vi "桶探测器值数据准备.vi"(0 "模块选择簇":T3, 5 "光源散斑簇":T2, 7 "图像簇":T1) -> (4 "照射差分求和数组":dbl[](array[numeric]), 6 "照射差分求和均值":dbl, 8 "优化光源散斑簇":T2, 10 "优化图像簇":T1)   [LabVIEW 2018]
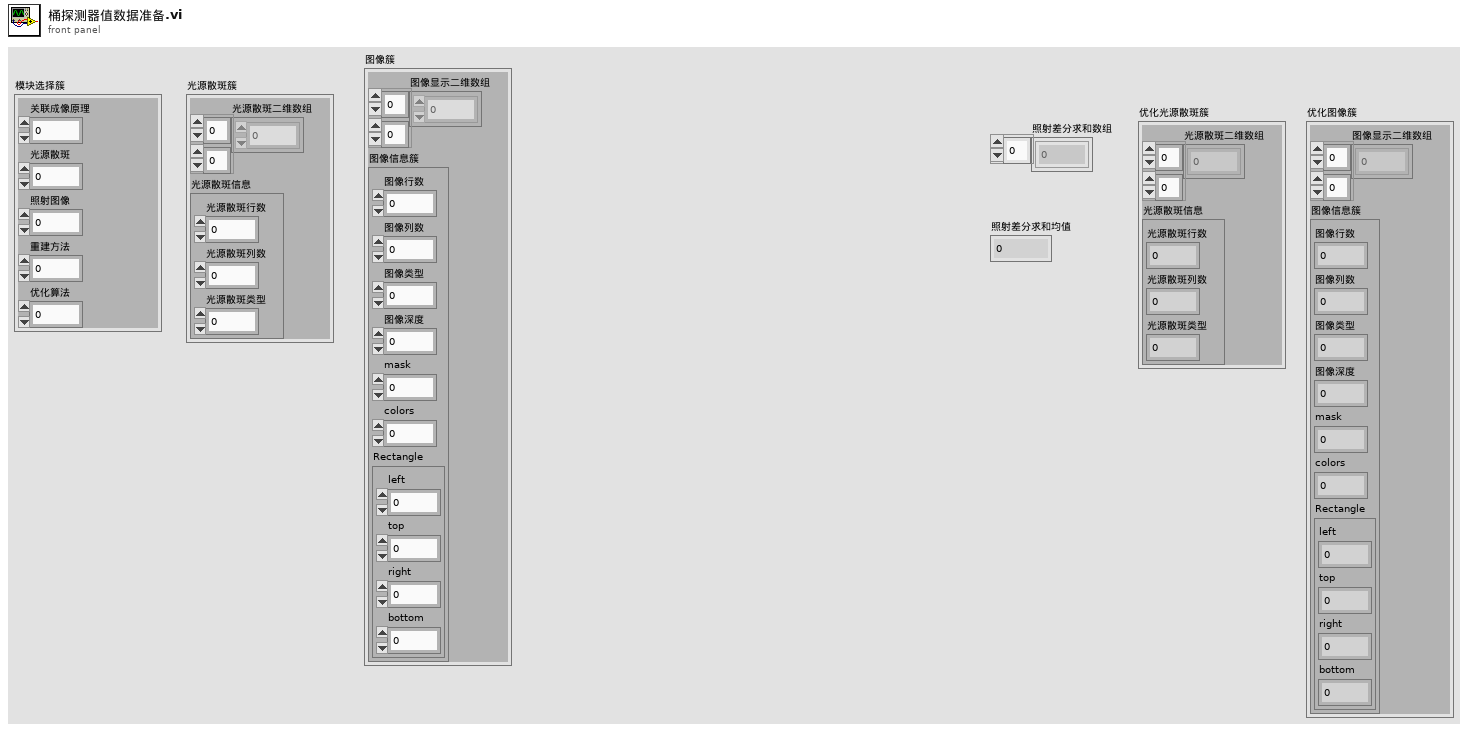
[diagram p1: front panel]
types:
  T1 = cluster{"图像显示二维数组":dbl[][], "图像信息簇":cluster{"图像行数":dbl, "图像列数":dbl, "图像类型":dbl, "图像深度":i32, "mask":i32, "colors":i32, "Rectangle":cluster{"left":i16, "top":i16, "right":i16, "bottom":i16}}}
  T2 = cluster{"光源散斑二维数组":dbl[][], "光源散斑信息":cluster{"光源散斑行数":dbl, "光源散斑列数":dbl, "光源散斑类型":dbl}}
  T3 = cluster{"关联成像原理":i32, "光源散斑":i32, "照射图像":i32, "重建方法":i32, "优化算法":i32}
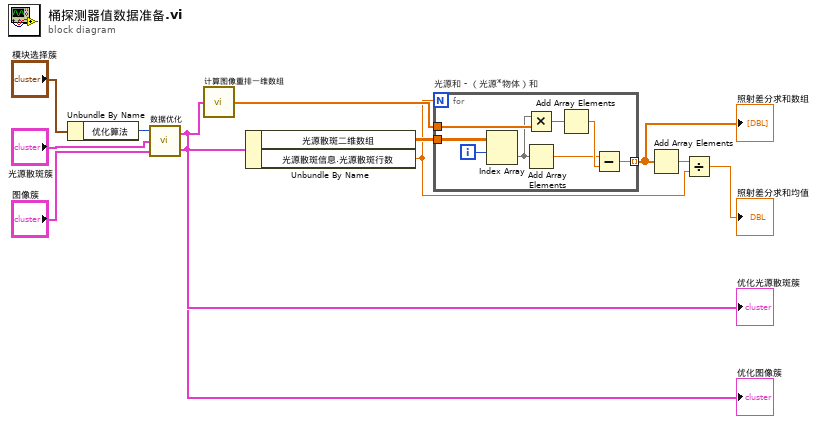
[diagram p0: block diagram]
diagram:
  n1 = Unbundle By Name("模块选择簇") -> ("优化算法"=w5:i32)
  n2 = call "数据优化.vi"("图像簇"="图像簇", "光源散斑簇"="光源散斑簇", "优化算法"=w5) -> ("优化光源散斑簇"=w2:T2, "优化图像簇"=w1:T1)
  "优化光源散斑簇" <- w2
  "优化图像簇" <- w1
  n3 = call "计算图像重排一维数组.vi"("优化图像簇"=w1) -> ("图像重排一维数组"=w12:dbl[])
  n4 = Unbundle By Name(w2) -> ("光源散斑二维数组"=w11:dbl[][], "光源散斑信息.光源散斑行数"=w8:dbl)
  n5 = for "光源和 - （光源*物体）和" {
    N: w8 -> [_]
    tunnel: w11 -> [w20]
    tunnel: w12 -> [w19]
    tunnel: [w15] -> w10 mode=indexing
    i -> [w14]
    n6 = Index Array(array=w20, index (row)=w14) -> (element=w17:dbl[])  [unwired: 1 in]
    n7 = Multiply(x=w17, y=w19) -> (x*y=w18:dbl[])
    n8 = Add Array Elements(numeric array=w17) -> (sum=w13:dbl)
    n9 = Add Array Elements(numeric array=w18) -> (sum=w16:dbl)
    n10 = Subtract(x=w13, y=w16) -> (x-y=w15:dbl)
  }
  "照射差分求和数组" <- w10
  n11 = Add Array Elements(numeric array=w10) -> (sum=w9:dbl)
  n12 = Divide(x=w9, y=w8) -> (x/y=→"照射差分求和均值":dbl)
